vi "WILT Step 3.vi"(7 "Station Number in":u32, 8 "Error In":errorcluster, 9 "Current Threshold":dbl=1.0 format="%#_13g", 10 "Step 3 Input":T1, 11 "Dryer Step 3 In":T3 {"Night Cycle Count" format="%04d"; "Day Cycle Count" format="%04d"}) -> (0 "Error Out":errorcluster, 2 "Step 3 Output":T1, 3 "Dryer Step 3 Output":T3 {"Night Cycle Count" format="%04d"; "Day Cycle Count" format="%04d"})   [LabVIEW 2016]
uses:
  Type Definitions/WILT Station Test State Cluster.ctl
  Type Definitions/WILT Dryer Test State.ctl
  Type Definitions/WILT Dryer.ctl
  Type Definitions/WILT Dryer Details.ctl
  Type Definitions/WILT Agilent Channel Definition.ctl
  Type Definitions/WILT DAQ Data.ctl
  Globals/WILT Globals Main Program.vi
panel:
  # "Day"
  # "Night"
  # "Day"
  # "Night"
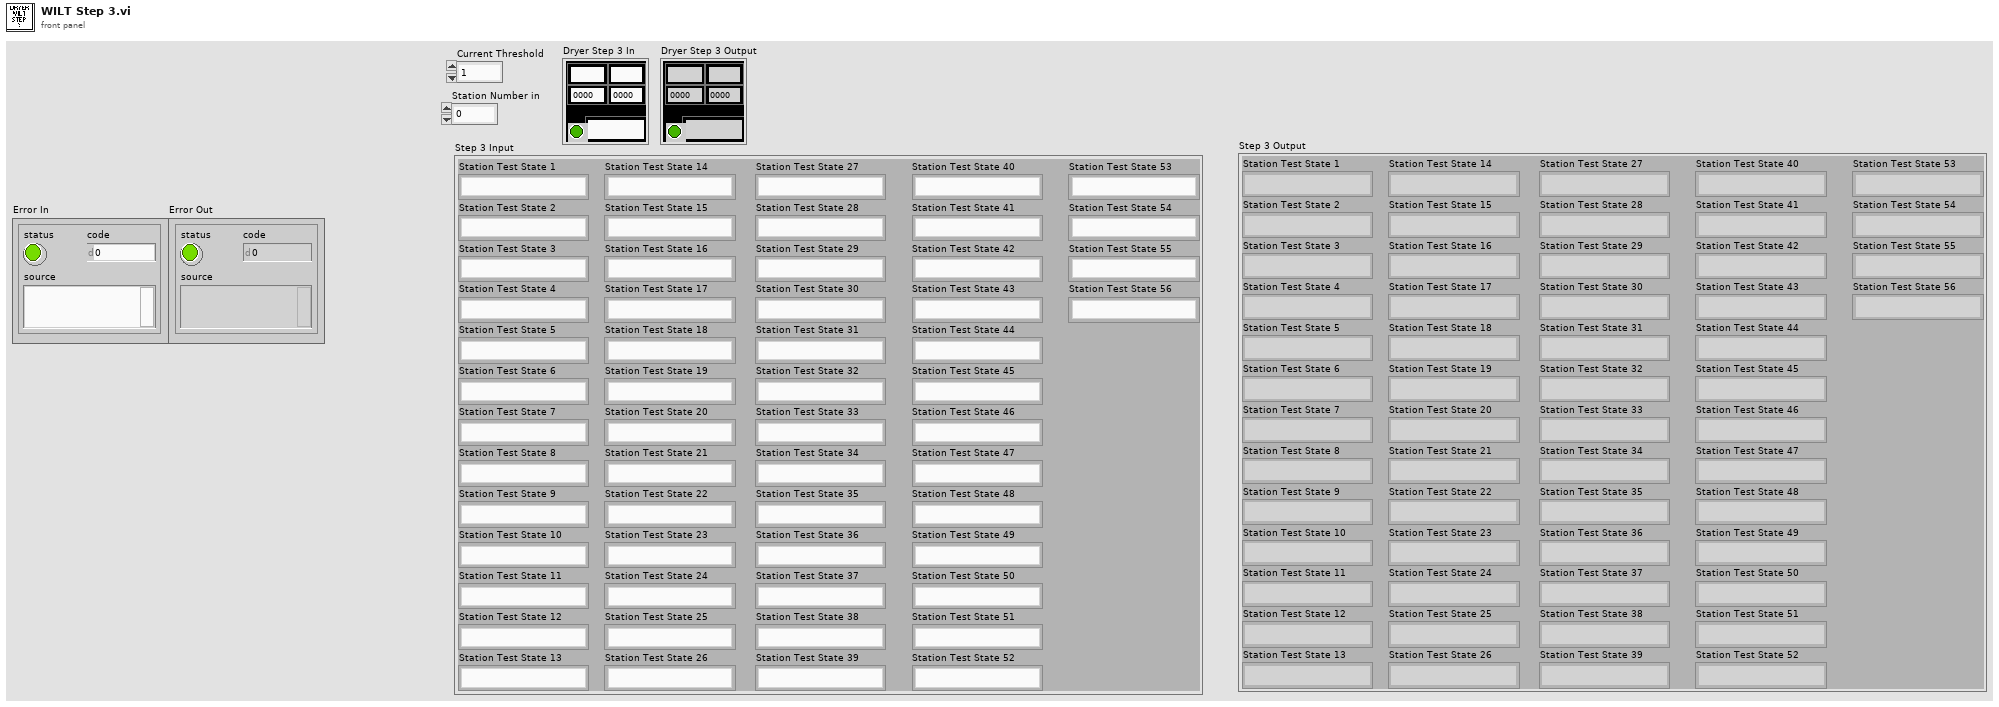
[diagram p1: front panel]
types:
  T1 = typedef "WILT Station Test State Cluster.ctl" = cluster{"Station Test State 1":T2, "Station Test State 2":T2, "Station Test State 3":T2, "Station Test State 4":T2, "Station Test State 5":T2, "Station Test State 6":T2, "Station Test State 7":T2, "Station Test State 8":T2, "Station Test State 9":T2, "Station Test State 10":T2, "Station Test State 11":T2, "Station Test State 12":T2, "Station Test State 13":T2, "Station Test State 14":T2, "Station Test State 15":T2, "Station Test State 16":T2, "Station Test State 17":T2, "Station Test State 18":T2, "Station Test State 19":T2, "Station Test State 20":T2, "Station Test State 21":T2, "Station Test State 22":T2, "Station Test State 23":T2, "Station Test State 24":T2, "Station Test State 25":T2, "Station Test State 26":T2, "Station Test State 27":T2, "Station Test State 28":T2, "Station Test State 29":T2, "Station Test State 30":T2, "Station Test State 31":T2, "Station Test State 32":T2, "Station Test State 33":T2, "Station Test State 34":T2, "Station Test State 35":T2, "Station Test State 36":T2, "Station Test State 37":T2, "Station Test State 38":T2, "Station Test State 39":T2, "Station Test State 40":T2, "Station Test State 41":T2, "Station Test State 42":T2, "Station Test State 43":T2, "Station Test State 44":T2, "Station Test State 45":T2, "Station Test State 46":T2, "Station Test State 47":T2, "Station Test State 48":T2, "Station Test State 49":T2, "Station Test State 50":T2, "Station Test State 51":T2, "Station Test State 52":T2, "Station Test State 53":T2, "Station Test State 54":T2, "Station Test State 55":T2, "Station Test State 56":T2}
  T2 = typedef "WILT Dryer Test State.ctl" = enum16{"No Serial Number", "Waiting for Dryer To Start", "Drying Clothes", "Water Injection 1 (On)", "Water Injection 1 Timer", "Water Injection 1 (Off)", "Pause Dryer", "Sending Start Stop CMD", "Pause Dryer 2", "Sending Start Stop CMD 2", "Drying Clothes 2", "Water Injection 2 (On)", "Water Injection 2 Timer", "Water Injection 2 (Off)", "Drying Clothes 3", "Cooling Down", "Sending Start Stop CMD 3", "Increment Cycle"}
  T3 = typedef "WILT Dryer.ctl" = cluster{"Lab ID":string, "Day Cycle Count":i32, "Station Label":string, "Dryer Details":T4, "Status Color":u32, "Invisible Button":bool, "Night Cycle Count":i32, "Station Index":i32, "Cycle Index":string, "Audit Alert":bool, "Agilent Channel Definition":T5, "DAQ Data":T6}
  T4 = typedef "WILT Dryer Details.ctl" = cluster{"Station":string, "Lab ID":string, "TR Number":string}
  T5 = typedef "WILT Agilent Channel Definition.ctl" = cluster{"Channel":string, "Station":string, "Label":string, "Agilent Station":string, "Data":dbl}
  T6 = typedef "WILT DAQ Data.ctl" = cluster{"L1 Current":dbl, "L2 Current":dbl, "Temperature  Deg F (TC)":dbl, "Volts":dbl, "Volts (208)":dbl, "SW (208)":dbl}
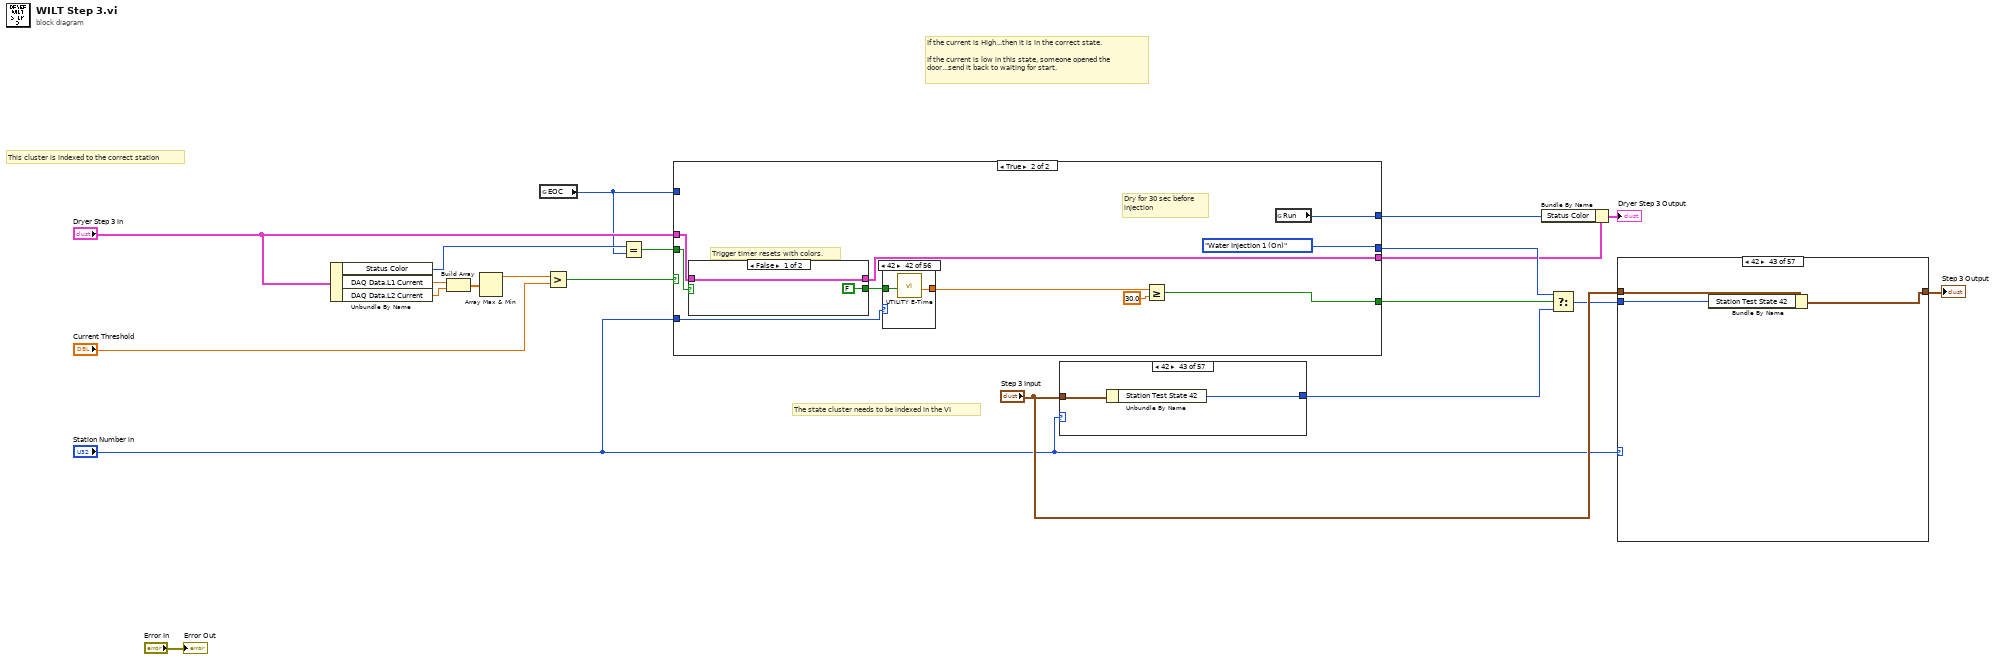
[diagram p0: block diagram]
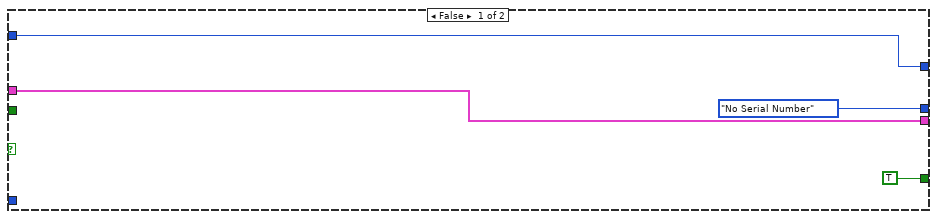
[diagram p2: hidden frame]
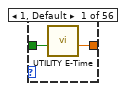
[diagram p3: hidden frame]
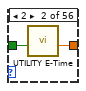
[diagram p4: hidden frame]
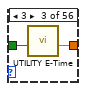
[diagram p5: hidden frame]
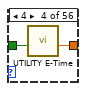
[diagram p6: hidden frame]
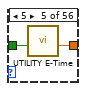
[diagram p7: hidden frame]
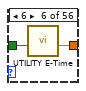
[diagram p8: hidden frame]
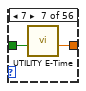
[diagram p9: hidden frame]
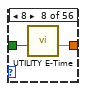
[diagram p10: hidden frame]
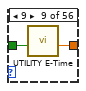
[diagram p11: hidden frame]
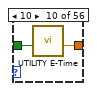
[diagram p12: hidden frame]
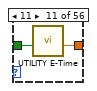
[diagram p13: hidden frame]
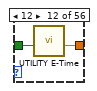
[diagram p14: hidden frame]
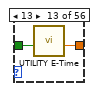
[diagram p15: hidden frame]
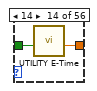
[diagram p16: hidden frame]
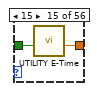
[diagram p17: hidden frame]
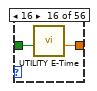
[diagram p18: hidden frame]
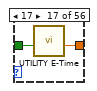
[diagram p19: hidden frame]
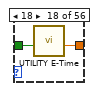
[diagram p20: hidden frame]
diagram:
  # "The state cluster needs to be indexed in the VI"
  # "This cluster is indexed to the correct station"
  # "If the current is High...then it is in the correct state.\n\nIf the current is low in this state, someone opened the \ndoor...send it back to waiting for start."
  n1 = Unbundle By Name("Dryer Step 3 In") -> ("Status Color"=w6:u32, "DAQ Data.L1 Current"=w10:dbl, "DAQ Data.L2 Current"=w9:dbl)
  n2 = Build Array(w10, w9) -> (w13:dbl[])
  n3 = Array Max & Min(array=w13) -> (max value=w11:dbl)  [unwired: 3 out]
  n4 = global read "WILT Globals Main Program.vi" "EOC"() -> (w1:u32)
  n5 = Greater?(x=w11, y="Current Threshold") -> (0:w8:bool)
  n6 = Equal?(x=w6, y=w1) -> (x = y?=w5:bool)
  n7 = case shown="True" w8 {
    tunnel: [TRUE w34] -> w20
    tunnel: "Station Number in" -> [_ w31]
    tunnel: "Dryer Step 3 In" -> [w22 w30]
    tunnel: [WILT_Dryer_Test_State."No Serial Number" ("Current State 2") WILT_Dryer_Test_State."Water Injection 1 (On)" ("Current State 2")] -> w7
    tunnel: w5 -> [_ w28]
    tunnel: [w22 w27] -> w3
    tunnel: [w23 w26] -> w2
    tunnel: w1 -> [w23 _]
    frame False {
    }
    frame True {
      # "Trigger timer resets with colors."
      # "Dry for 30 sec before\ninjection"
      n8 = case shown="False" w28 {
        tunnel: [FALSE TRUE] -> w32
        tunnel: w30 -> [w148 w150]
        tunnel: [w148 w150] -> w27
        frame False {
        }
        frame True {
        }
      }
      n9 = case shown="42" w31 {
        tunnel: [w37 w38 w40 w42 w44 w46 w48 w50 w52 w54 w56 w58 w60 w62 w64 w66 w68 w70 w72 w74 w76 w78 w80 w82 w84 w86 w88 w90 w92 w94 w96 w98 w100 w102 w104 w106 w108 w110 w112 w114 w116 w118 w120 w122 w124 w126 w128 w130 w132 w134 w136 w138 w140 w142 w144 w146] -> w33
        tunnel: w32 -> [w36 w39 w41 w43 w45 w47 w49 w51 w53 w55 w57 w59 w61 w63 w65 w67 w69 w71 w73 w75 w77 w79 w81 w83 w85 w87 w89 w91 w93 w95 w97 w99 w101 w103 w105 w107 w109 w111 w113 w115 w117 w119 w121 w123 w125 w127 w129 w131 w133 w135 w137 w139 w141 w143 w145 w147]
        frame 1, Default {
          n10 = call "UTILITY E-Time.vi"("Reset"=w36) -> ("Elapsed Time (sec)"=w37:dbl)  [unwired: 8 in, 2 out]
        }
        frame 2 {
          n11 = call "UTILITY E-Time.vi"("Reset"=w39) -> ("Elapsed Time (sec)"=w38:dbl)  [unwired: 8 in, 2 out]
        }
        frame 3 {
          n12 = call "UTILITY E-Time.vi"("Reset"=w41) -> ("Elapsed Time (sec)"=w40:dbl)  [unwired: 8 in, 2 out]
        }
        frame 4 {
          n13 = call "UTILITY E-Time.vi"("Reset"=w43) -> ("Elapsed Time (sec)"=w42:dbl)  [unwired: 8 in, 2 out]
        }
        frame 5 {
          n14 = call "UTILITY E-Time.vi"("Reset"=w45) -> ("Elapsed Time (sec)"=w44:dbl)  [unwired: 8 in, 2 out]
        }
        frame 6 {
          n15 = call "UTILITY E-Time.vi"("Reset"=w47) -> ("Elapsed Time (sec)"=w46:dbl)  [unwired: 8 in, 2 out]
        }
        frame 7 {
          n16 = call "UTILITY E-Time.vi"("Reset"=w49) -> ("Elapsed Time (sec)"=w48:dbl)  [unwired: 8 in, 2 out]
        }
        frame 8 {
          n17 = call "UTILITY E-Time.vi"("Reset"=w51) -> ("Elapsed Time (sec)"=w50:dbl)  [unwired: 8 in, 2 out]
        }
        frame 9 {
          n18 = call "UTILITY E-Time.vi"("Reset"=w53) -> ("Elapsed Time (sec)"=w52:dbl)  [unwired: 8 in, 2 out]
        }
        frame 10 {
          n19 = call "UTILITY E-Time.vi"("Reset"=w55) -> ("Elapsed Time (sec)"=w54:dbl)  [unwired: 8 in, 2 out]
        }
        frame 11 {
          n20 = call "UTILITY E-Time.vi"("Reset"=w57) -> ("Elapsed Time (sec)"=w56:dbl)  [unwired: 8 in, 2 out]
        }
        frame 12 {
          n21 = call "UTILITY E-Time.vi"("Reset"=w59) -> ("Elapsed Time (sec)"=w58:dbl)  [unwired: 8 in, 2 out]
        }
        frame 13 {
          n22 = call "UTILITY E-Time.vi"("Reset"=w61) -> ("Elapsed Time (sec)"=w60:dbl)  [unwired: 8 in, 2 out]
        }
        frame 14 {
          n23 = call "UTILITY E-Time.vi"("Reset"=w63) -> ("Elapsed Time (sec)"=w62:dbl)  [unwired: 8 in, 2 out]
        }
        frame 15 {
          n24 = call "UTILITY E-Time.vi"("Reset"=w65) -> ("Elapsed Time (sec)"=w64:dbl)  [unwired: 8 in, 2 out]
        }
        frame 16 {
          n25 = call "UTILITY E-Time.vi"("Reset"=w67) -> ("Elapsed Time (sec)"=w66:dbl)  [unwired: 8 in, 2 out]
        }
        frame 17 {
          n26 = call "UTILITY E-Time.vi"("Reset"=w69) -> ("Elapsed Time (sec)"=w68:dbl)  [unwired: 8 in, 2 out]
        }
        frame 18 {
          n27 = call "UTILITY E-Time.vi"("Reset"=w71) -> ("Elapsed Time (sec)"=w70:dbl)  [unwired: 8 in, 2 out]
        }
        frame 19 {
          n28 = call "UTILITY E-Time.vi"("Reset"=w73) -> ("Elapsed Time (sec)"=w72:dbl)  [unwired: 8 in, 2 out]
        }
        frame 20 {
          n29 = call "UTILITY E-Time.vi"("Reset"=w75) -> ("Elapsed Time (sec)"=w74:dbl)  [unwired: 8 in, 2 out]
        }
        frame 21 {
          n30 = call "UTILITY E-Time.vi"("Reset"=w77) -> ("Elapsed Time (sec)"=w76:dbl)  [unwired: 8 in, 2 out]
        }
        frame 22 {
          n31 = call "UTILITY E-Time.vi"("Reset"=w79) -> ("Elapsed Time (sec)"=w78:dbl)  [unwired: 8 in, 2 out]
        }
        frame 23 {
          n32 = call "UTILITY E-Time.vi"("Reset"=w81) -> ("Elapsed Time (sec)"=w80:dbl)  [unwired: 8 in, 2 out]
        }
        frame 24 {
          n33 = call "UTILITY E-Time.vi"("Reset"=w83) -> ("Elapsed Time (sec)"=w82:dbl)  [unwired: 8 in, 2 out]
        }
        frame 25 {
          n34 = call "UTILITY E-Time.vi"("Reset"=w85) -> ("Elapsed Time (sec)"=w84:dbl)  [unwired: 8 in, 2 out]
        }
        frame 26 {
          n35 = call "UTILITY E-Time.vi"("Reset"=w87) -> ("Elapsed Time (sec)"=w86:dbl)  [unwired: 8 in, 2 out]
        }
        frame 27 {
          n36 = call "UTILITY E-Time.vi"("Reset"=w89) -> ("Elapsed Time (sec)"=w88:dbl)  [unwired: 8 in, 2 out]
        }
        frame 28 {
          n37 = call "UTILITY E-Time.vi"("Reset"=w91) -> ("Elapsed Time (sec)"=w90:dbl)  [unwired: 8 in, 2 out]
        }
        frame 29 {
          n38 = call "UTILITY E-Time.vi"("Reset"=w93) -> ("Elapsed Time (sec)"=w92:dbl)  [unwired: 8 in, 2 out]
        }
        frame 30 {
          n39 = call "UTILITY E-Time.vi"("Reset"=w95) -> ("Elapsed Time (sec)"=w94:dbl)  [unwired: 8 in, 2 out]
        }
        frame 31 {
          n40 = call "UTILITY E-Time.vi"("Reset"=w97) -> ("Elapsed Time (sec)"=w96:dbl)  [unwired: 8 in, 2 out]
        }
        frame 32 {
          n41 = call "UTILITY E-Time.vi"("Reset"=w99) -> ("Elapsed Time (sec)"=w98:dbl)  [unwired: 8 in, 2 out]
        }
        frame 33 {
          n42 = call "UTILITY E-Time.vi"("Reset"=w101) -> ("Elapsed Time (sec)"=w100:dbl)  [unwired: 8 in, 2 out]
        }
        frame 34 {
          n43 = call "UTILITY E-Time.vi"("Reset"=w103) -> ("Elapsed Time (sec)"=w102:dbl)  [unwired: 8 in, 2 out]
        }
        frame 35 {
          n44 = call "UTILITY E-Time.vi"("Reset"=w105) -> ("Elapsed Time (sec)"=w104:dbl)  [unwired: 8 in, 2 out]
        }
        frame 36 {
          n45 = call "UTILITY E-Time.vi"("Reset"=w107) -> ("Elapsed Time (sec)"=w106:dbl)  [unwired: 8 in, 2 out]
        }
        frame 37 {
          n46 = call "UTILITY E-Time.vi"("Reset"=w109) -> ("Elapsed Time (sec)"=w108:dbl)  [unwired: 8 in, 2 out]
        }
        frame 38 {
          n47 = call "UTILITY E-Time.vi"("Reset"=w111) -> ("Elapsed Time (sec)"=w110:dbl)  [unwired: 8 in, 2 out]
        }
        frame 39 {
          n48 = call "UTILITY E-Time.vi"("Reset"=w113) -> ("Elapsed Time (sec)"=w112:dbl)  [unwired: 8 in, 2 out]
        }
        frame 40 {
          n49 = call "UTILITY E-Time.vi"("Reset"=w115) -> ("Elapsed Time (sec)"=w114:dbl)  [unwired: 8 in, 2 out]
        }
        frame 41 {
          n50 = call "UTILITY E-Time.vi"("Reset"=w117) -> ("Elapsed Time (sec)"=w116:dbl)  [unwired: 8 in, 2 out]
        }
        frame 42 {
          n51 = call "UTILITY E-Time.vi"("Reset"=w119) -> ("Elapsed Time (sec)"=w118:dbl)  [unwired: 8 in, 2 out]
        }
        frame 43 {
          n52 = call "UTILITY E-Time.vi"("Reset"=w121) -> ("Elapsed Time (sec)"=w120:dbl)  [unwired: 8 in, 2 out]
        }
        frame 44 {
          n53 = call "UTILITY E-Time.vi"("Reset"=w123) -> ("Elapsed Time (sec)"=w122:dbl)  [unwired: 8 in, 2 out]
        }
        frame 45 {
          n54 = call "UTILITY E-Time.vi"("Reset"=w125) -> ("Elapsed Time (sec)"=w124:dbl)  [unwired: 8 in, 2 out]
        }
        frame 46 {
          n55 = call "UTILITY E-Time.vi"("Reset"=w127) -> ("Elapsed Time (sec)"=w126:dbl)  [unwired: 8 in, 2 out]
        }
        frame 47 {
          n56 = call "UTILITY E-Time.vi"("Reset"=w129) -> ("Elapsed Time (sec)"=w128:dbl)  [unwired: 8 in, 2 out]
        }
        frame 48 {
          n57 = call "UTILITY E-Time.vi"("Reset"=w131) -> ("Elapsed Time (sec)"=w130:dbl)  [unwired: 8 in, 2 out]
        }
        frame 49 {
          n58 = call "UTILITY E-Time.vi"("Reset"=w133) -> ("Elapsed Time (sec)"=w132:dbl)  [unwired: 8 in, 2 out]
        }
        frame 50 {
          n59 = call "UTILITY E-Time.vi"("Reset"=w135) -> ("Elapsed Time (sec)"=w134:dbl)  [unwired: 8 in, 2 out]
        }
        frame 51 {
          n60 = call "UTILITY E-Time.vi"("Reset"=w137) -> ("Elapsed Time (sec)"=w136:dbl)  [unwired: 8 in, 2 out]
        }
        frame 52 {
          n61 = call "UTILITY E-Time.vi"("Reset"=w139) -> ("Elapsed Time (sec)"=w138:dbl)  [unwired: 8 in, 2 out]
        }
        frame 53 {
          n62 = call "UTILITY E-Time.vi"("Reset"=w141) -> ("Elapsed Time (sec)"=w140:dbl)  [unwired: 8 in, 2 out]
        }
        frame 54 {
          n63 = call "UTILITY E-Time.vi"("Reset"=w143) -> ("Elapsed Time (sec)"=w142:dbl)  [unwired: 8 in, 2 out]
        }
        frame 55 {
          n64 = call "UTILITY E-Time.vi"("Reset"=w145) -> ("Elapsed Time (sec)"=w144:dbl)  [unwired: 8 in, 2 out]
        }
        frame 56 {
          n65 = call "UTILITY E-Time.vi"("Reset"=w147) -> ("Elapsed Time (sec)"=w146:dbl)  [unwired: 8 in, 2 out]
        }
      }
      n66 = Greater Or Equal?(x=w33, y=30.0) -> (x >= y?=w34:bool)
      n67 = global read "WILT Globals Main Program.vi" "Run"() -> (w26:u32)
    }
  }
  n68 = case shown="42" "Station Number in" {
    tunnel: "Step 3 Input" -> [_ w154 w156 w158 w160 w162 w164 w166 w168 w170 w172 w174 w176 w178 w180 w182 w184 w186 w188 w190 w192 w194 w196 w198 w200 w202 w204 w206 w208 w210 w212 w214 w216 w218 w220 w222 w224 w226 w228 w230 w232 w234 w236 w238 w240 w242 w244 w246 w248 w250 w252 w254 w256 w258 w260 w262 w264]
    tunnel: [WILT_Dryer_Test_State."No Serial Number" ("Station Test State 56") w153 w155 w157 w159 w161 w163 w165 w167 w169 w171 w173 w175 w177 w179 w181 w183 w185 w187 w189 w191 w193 w195 w197 w199 w201 w203 w205 w207 w209 w211 w213 w215 w217 w219 w221 w223 w225 w227 w229 w231 w233 w235 w237 w239 w241 w243 w245 w247 w249 w251 w253 w255 w257 w259 w261 w263] -> w17
    frame 0, Default {
      # "This is not a station.\nDo nothing"
    }
    frame 1 {
      n69 = Unbundle By Name(w154) -> ("Station Test State 1"=w153:T2)
    }
    frame 2 {
      n70 = Unbundle By Name(w156) -> ("Station Test State 2"=w155:T2)
    }
    frame 3 {
      n71 = Unbundle By Name(w158) -> ("Station Test State 3"=w157:T2)
    }
    frame 4 {
      n72 = Unbundle By Name(w160) -> ("Station Test State 4"=w159:T2)
    }
    frame 5 {
      n73 = Unbundle By Name(w162) -> ("Station Test State 5"=w161:T2)
    }
    frame 6 {
      n74 = Unbundle By Name(w164) -> ("Station Test State 6"=w163:T2)
    }
    frame 7 {
      n75 = Unbundle By Name(w166) -> ("Station Test State 7"=w165:T2)
    }
    frame 8 {
      n76 = Unbundle By Name(w168) -> ("Station Test State 8"=w167:T2)
    }
    frame 9 {
      n77 = Unbundle By Name(w170) -> ("Station Test State 9"=w169:T2)
    }
    frame 10 {
      n78 = Unbundle By Name(w172) -> ("Station Test State 10"=w171:T2)
    }
    frame 11 {
      n79 = Unbundle By Name(w174) -> ("Station Test State 11"=w173:T2)
    }
    frame 12 {
      n80 = Unbundle By Name(w176) -> ("Station Test State 12"=w175:T2)
    }
    frame 13 {
      n81 = Unbundle By Name(w178) -> ("Station Test State 13"=w177:T2)
    }
    frame 14 {
      n82 = Unbundle By Name(w180) -> ("Station Test State 14"=w179:T2)
    }
    frame 15 {
      n83 = Unbundle By Name(w182) -> ("Station Test State 15"=w181:T2)
    }
    frame 16 {
      n84 = Unbundle By Name(w184) -> ("Station Test State 16"=w183:T2)
    }
    frame 17 {
      n85 = Unbundle By Name(w186) -> ("Station Test State 17"=w185:T2)
    }
    frame 18 {
      n86 = Unbundle By Name(w188) -> ("Station Test State 18"=w187:T2)
    }
    frame 19 {
      n87 = Unbundle By Name(w190) -> ("Station Test State 19"=w189:T2)
    }
    frame 20 {
      n88 = Unbundle By Name(w192) -> ("Station Test State 20"=w191:T2)
    }
    frame 21 {
      n89 = Unbundle By Name(w194) -> ("Station Test State 21"=w193:T2)
    }
    frame 22 {
      n90 = Unbundle By Name(w196) -> ("Station Test State 22"=w195:T2)
    }
    frame 23 {
      n91 = Unbundle By Name(w198) -> ("Station Test State 23"=w197:T2)
    }
    frame 24 {
      n92 = Unbundle By Name(w200) -> ("Station Test State 24"=w199:T2)
    }
    frame 25 {
      n93 = Unbundle By Name(w202) -> ("Station Test State 25"=w201:T2)
    }
    frame 26 {
      n94 = Unbundle By Name(w204) -> ("Station Test State 26"=w203:T2)
    }
    frame 27 {
      n95 = Unbundle By Name(w206) -> ("Station Test State 27"=w205:T2)
    }
    frame 28 {
      n96 = Unbundle By Name(w208) -> ("Station Test State 28"=w207:T2)
    }
    frame 29 {
      n97 = Unbundle By Name(w210) -> ("Station Test State 29"=w209:T2)
    }
    frame 30 {
      n98 = Unbundle By Name(w212) -> ("Station Test State 30"=w211:T2)
    }
    frame 31 {
      n99 = Unbundle By Name(w214) -> ("Station Test State 31"=w213:T2)
    }
    frame 32 {
      n100 = Unbundle By Name(w216) -> ("Station Test State 32"=w215:T2)
    }
    frame 33 {
      n101 = Unbundle By Name(w218) -> ("Station Test State 33"=w217:T2)
    }
    frame 34 {
      n102 = Unbundle By Name(w220) -> ("Station Test State 34"=w219:T2)
    }
    frame 35 {
      n103 = Unbundle By Name(w222) -> ("Station Test State 35"=w221:T2)
    }
    frame 36 {
      n104 = Unbundle By Name(w224) -> ("Station Test State 36"=w223:T2)
    }
    frame 37 {
      n105 = Unbundle By Name(w226) -> ("Station Test State 37"=w225:T2)
    }
    frame 38 {
      n106 = Unbundle By Name(w228) -> ("Station Test State 38"=w227:T2)
    }
    frame 39 {
      n107 = Unbundle By Name(w230) -> ("Station Test State 39"=w229:T2)
    }
    frame 40 {
      n108 = Unbundle By Name(w232) -> ("Station Test State 40"=w231:T2)
    }
    frame 41 {
      n109 = Unbundle By Name(w234) -> ("Station Test State 41"=w233:T2)
    }
    frame 42 {
      n110 = Unbundle By Name(w236) -> ("Station Test State 42"=w235:T2)
    }
    frame 43 {
      n111 = Unbundle By Name(w238) -> ("Station Test State 43"=w237:T2)
    }
    frame 44 {
      n112 = Unbundle By Name(w240) -> ("Station Test State 44"=w239:T2)
    }
    frame 45 {
      n113 = Unbundle By Name(w242) -> ("Station Test State 45"=w241:T2)
    }
    frame 46 {
      n114 = Unbundle By Name(w244) -> ("Station Test State 46"=w243:T2)
    }
    frame 47 {
      n115 = Unbundle By Name(w246) -> ("Station Test State 47"=w245:T2)
    }
    frame 48 {
      n116 = Unbundle By Name(w248) -> ("Station Test State 48"=w247:T2)
    }
    frame 49 {
      n117 = Unbundle By Name(w250) -> ("Station Test State 49"=w249:T2)
    }
    frame 50 {
      n118 = Unbundle By Name(w252) -> ("Station Test State 50"=w251:T2)
    }
    frame 51 {
      n119 = Unbundle By Name(w254) -> ("Station Test State 51"=w253:T2)
    }
    frame 52 {
      n120 = Unbundle By Name(w256) -> ("Station Test State 52"=w255:T2)
    }
    frame 53 {
      n121 = Unbundle By Name(w258) -> ("Station Test State 53"=w257:T2)
    }
    frame 54 {
      n122 = Unbundle By Name(w260) -> ("Station Test State 54"=w259:T2)
    }
    frame 55 {
      n123 = Unbundle By Name(w262) -> ("Station Test State 55"=w261:T2)
    }
    frame 56 {
      n124 = Unbundle By Name(w264) -> ("Station Test State 56"=w263:T2)
    }
  }
  n125 = Bundle By Name(cluster=w3, "Status Color"=w2) -> (→"Dryer Step 3 Output":T3)
  n126 = Select(t=w7, s=w20, f=w17) -> (s? t:f=w16:T2)
  n127 = case shown="42" "Station Number in" {
    tunnel: "Step 3 Input" -> [w265 w268 w271 w274 w277 w280 w283 w286 w289 w292 w295 w298 w301 w304 w307 w310 w313 w316 w319 w322 w325 w328 w331 w334 w337 w340 w343 w346 w349 w352 w355 w358 w361 w364 w367 w370 w373 w376 w379 w382 w385 w388 w391 w394 w397 w400 w403 w406 w409 w412 w415 w418 w421 w424 w427 w430 w433]
    tunnel: w16 -> [_ w267 w269 w272 w275 w278 w281 w284 w287 w290 w293 w296 w299 w302 w305 w308 w311 w314 w317 w320 w323 w326 w329 w332 w335 w338 w341 w344 w347 w350 w353 w356 w359 w362 w365 w368 w371 w374 w377 w380 w383 w386 w389 w392 w395 w398 w401 w404 w407 w410 w413 w416 w419 w422 w425 w428 w431]
    tunnel: [w265 w266 w270 w273 w276 w279 w282 w285 w288 w291 w294 w297 w300 w303 w306 w309 w312 w315 w318 w321 w324 w327 w330 w333 w336 w339 w342 w345 w348 w351 w354 w357 w360 w363 w366 w369 w372 w375 w378 w381 w384 w387 w390 w393 w396 w399 w402 w405 w408 w411 w414 w417 w420 w423 w426 w429 w432] -> w19
    frame 0, Default {
      # "Not a valid station. Do nothing"
    }
    frame 1 {
      n128 = Bundle By Name(cluster=w268, "Station Test State 1"=w267) -> (w266:T1)
    }
    frame 2 {
      n129 = Bundle By Name(cluster=w271, "Station Test State 2"=w269) -> (w270:T1)
    }
    frame 3 {
      n130 = Bundle By Name(cluster=w274, "Station Test State 3"=w272) -> (w273:T1)
    }
    frame 4 {
      n131 = Bundle By Name(cluster=w277, "Station Test State 4"=w275) -> (w276:T1)
    }
    frame 5 {
      n132 = Bundle By Name(cluster=w280, "Station Test State 5"=w278) -> (w279:T1)
    }
    frame 6 {
      n133 = Bundle By Name(cluster=w283, "Station Test State 6"=w281) -> (w282:T1)
    }
    frame 7 {
      n134 = Bundle By Name(cluster=w286, "Station Test State 7"=w284) -> (w285:T1)
    }
    frame 8 {
      n135 = Bundle By Name(cluster=w289, "Station Test State 8"=w287) -> (w288:T1)
    }
    frame 9 {
      n136 = Bundle By Name(cluster=w292, "Station Test State 9"=w290) -> (w291:T1)
    }
    frame 10 {
      n137 = Bundle By Name(cluster=w295, "Station Test State 10"=w293) -> (w294:T1)
    }
    frame 11 {
      n138 = Bundle By Name(cluster=w298, "Station Test State 11"=w296) -> (w297:T1)
    }
    frame 12 {
      n139 = Bundle By Name(cluster=w301, "Station Test State 12"=w299) -> (w300:T1)
    }
    frame 13 {
      n140 = Bundle By Name(cluster=w304, "Station Test State 13"=w302) -> (w303:T1)
    }
    frame 14 {
      n141 = Bundle By Name(cluster=w307, "Station Test State 14"=w305) -> (w306:T1)
    }
    frame 15 {
      n142 = Bundle By Name(cluster=w310, "Station Test State 15"=w308) -> (w309:T1)
    }
    frame 16 {
      n143 = Bundle By Name(cluster=w313, "Station Test State 16"=w311) -> (w312:T1)
    }
    frame 17 {
      n144 = Bundle By Name(cluster=w316, "Station Test State 17"=w314) -> (w315:T1)
    }
    frame 18 {
      n145 = Bundle By Name(cluster=w319, "Station Test State 18"=w317) -> (w318:T1)
    }
    frame 19 {
      n146 = Bundle By Name(cluster=w322, "Station Test State 19"=w320) -> (w321:T1)
    }
    frame 20 {
      n147 = Bundle By Name(cluster=w325, "Station Test State 20"=w323) -> (w324:T1)
    }
    frame 21 {
      n148 = Bundle By Name(cluster=w328, "Station Test State 21"=w326) -> (w327:T1)
    }
    frame 22 {
      n149 = Bundle By Name(cluster=w331, "Station Test State 22"=w329) -> (w330:T1)
    }
    frame 23 {
      n150 = Bundle By Name(cluster=w334, "Station Test State 23"=w332) -> (w333:T1)
    }
    frame 24 {
      n151 = Bundle By Name(cluster=w337, "Station Test State 24"=w335) -> (w336:T1)
    }
    frame 25 {
      n152 = Bundle By Name(cluster=w340, "Station Test State 25"=w338) -> (w339:T1)
    }
    frame 26 {
      n153 = Bundle By Name(cluster=w343, "Station Test State 26"=w341) -> (w342:T1)
    }
    frame 27 {
      n154 = Bundle By Name(cluster=w346, "Station Test State 27"=w344) -> (w345:T1)
    }
    frame 28 {
      n155 = Bundle By Name(cluster=w349, "Station Test State 28"=w347) -> (w348:T1)
    }
    frame 29 {
      n156 = Bundle By Name(cluster=w352, "Station Test State 29"=w350) -> (w351:T1)
    }
    frame 30 {
      n157 = Bundle By Name(cluster=w355, "Station Test State 30"=w353) -> (w354:T1)
    }
    frame 31 {
      n158 = Bundle By Name(cluster=w358, "Station Test State 31"=w356) -> (w357:T1)
    }
    frame 32 {
      n159 = Bundle By Name(cluster=w361, "Station Test State 32"=w359) -> (w360:T1)
    }
    frame 33 {
      n160 = Bundle By Name(cluster=w364, "Station Test State 33"=w362) -> (w363:T1)
    }
    frame 34 {
      n161 = Bundle By Name(cluster=w367, "Station Test State 34"=w365) -> (w366:T1)
    }
    frame 35 {
      n162 = Bundle By Name(cluster=w370, "Station Test State 35"=w368) -> (w369:T1)
    }
    frame 36 {
      n163 = Bundle By Name(cluster=w373, "Station Test State 36"=w371) -> (w372:T1)
    }
    frame 37 {
      n164 = Bundle By Name(cluster=w376, "Station Test State 37"=w374) -> (w375:T1)
    }
    frame 38 {
      n165 = Bundle By Name(cluster=w379, "Station Test State 38"=w377) -> (w378:T1)
    }
    frame 39 {
      n166 = Bundle By Name(cluster=w382, "Station Test State 39"=w380) -> (w381:T1)
    }
    frame 40 {
      n167 = Bundle By Name(cluster=w385, "Station Test State 40"=w383) -> (w384:T1)
    }
    frame 41 {
      n168 = Bundle By Name(cluster=w388, "Station Test State 41"=w386) -> (w387:T1)
    }
    frame 42 {
      n169 = Bundle By Name(cluster=w391, "Station Test State 42"=w389) -> (w390:T1)
    }
    frame 43 {
      n170 = Bundle By Name(cluster=w394, "Station Test State 43"=w392) -> (w393:T1)
    }
    frame 44 {
      n171 = Bundle By Name(cluster=w397, "Station Test State 44"=w395) -> (w396:T1)
    }
    frame 45 {
      n172 = Bundle By Name(cluster=w400, "Station Test State 45"=w398) -> (w399:T1)
    }
    frame 46 {
      n173 = Bundle By Name(cluster=w403, "Station Test State 46"=w401) -> (w402:T1)
    }
    frame 47 {
      n174 = Bundle By Name(cluster=w406, "Station Test State 47"=w404) -> (w405:T1)
    }
    frame 48 {
      n175 = Bundle By Name(cluster=w409, "Station Test State 48"=w407) -> (w408:T1)
    }
    frame 49 {
      n176 = Bundle By Name(cluster=w412, "Station Test State 49"=w410) -> (w411:T1)
    }
    frame 50 {
      n177 = Bundle By Name(cluster=w415, "Station Test State 50"=w413) -> (w414:T1)
    }
    frame 51 {
      n178 = Bundle By Name(cluster=w418, "Station Test State 51"=w416) -> (w417:T1)
    }
    frame 52 {
      n179 = Bundle By Name(cluster=w421, "Station Test State 52"=w419) -> (w420:T1)
    }
    frame 53 {
      n180 = Bundle By Name(cluster=w424, "Station Test State 53"=w422) -> (w423:T1)
    }
    frame 54 {
      n181 = Bundle By Name(cluster=w427, "Station Test State 54"=w425) -> (w426:T1)
    }
    frame 55 {
      n182 = Bundle By Name(cluster=w430, "Station Test State 55"=w428) -> (w429:T1)
    }
    frame 56 {
      n183 = Bundle By Name(cluster=w433, "Station Test State 56"=w431) -> (w432:T1)
    }
  }
  "Step 3 Output" <- w19
  "Error Out" <- "Error In"
